vi "DRIVE_SPEED_CONTROL.vi"(4 "Time_Seconds":dbl, 5 "Speed PID":T2, 6 "Speed (PV)":dbl, 7 "SIMPLE_MOTOR_FF":T1 {"KnInv" format="%13.4f"; "Ka" format="%13.4f"; "Kv" format="%13.4f"; "Ks" format="%13.4f"}, 9 "Speed Target (SP)":dbl, 10 "Max SP Rate":dbl, 11 "Max Speed Ft/Sec":dbl) -> (0 "FeedForward":dbl, 1 "SpeedDmdAccel":dbl, 2 "SpeedDmd":dbl, 3 "CO-ControlOutput":dbl)   [LabVIEW 2019]
uses:
  DRIVE_PID_TUNING.ctl
  <vilib>/Rock Robotics/WPI/ThirdParty/JAS_Junk/TrajLib/TypeDef/SIMPLE_MOTOR_FF.ctl
  <vilib>/Rock Robotics/WPI/ThirdParty/JAS_Junk/TrajLib/SlewRateLimiter_New.vi
  <vilib>/Rock Robotics/WPI/ThirdParty/JAS_Junk/TrajLib/SlewRateLimiter_Reset.vi
  <vilib>/Rock Robotics/WPI/ThirdParty/JAS_Junk/TrajLib/SlewRateLimiter_Calculate.vi
  <vilib>/Rock Robotics/WPI/ThirdParty/JAS_Junk/TrajLib/SlewRateLimiter_SetRate.vi
  <vilib>/Rock Robotics/WPI/ThirdParty/JAS_Junk/TrajLib/PIDController_AtSetpoint.vi
  <vilib>/Rock Robotics/WPI/ThirdParty/JAS_Junk/TrajLib/PIDController_SetPIDF.vi
  <vilib>/Rock Robotics/WPI/ThirdParty/JAS_Junk/TrajLib/PIDController_SetDerivativeFilter.vi
  <vilib>/Rock Robotics/WPI/ThirdParty/JAS_Junk/TrajLib/PIDController_SetIntegratorRange.vi
  <vilib>/Rock Robotics/WPI/ThirdParty/JAS_Junk/TrajLib/PIDController_SetTolerancePandV.vi
  <vilib>/Rock Robotics/WPI/ThirdParty/JAS_Junk/TrajLib/PIDController_DisableContinousInput.vi
  <vilib>/Rock Robotics/WPI/ThirdParty/JAS_Junk/TrajLib/PIDController_EnableContinousInput.vi
  <vilib>/Rock Robotics/WPI/ThirdParty/JAS_Junk/TrajLib/PIDController_Reset.vi
  <vilib>/Rock Robotics/WPI/ThirdParty/JAS_Junk/TrajLib/PIDController_New.vi
  <vilib>/Rock Robotics/WPI/ThirdParty/JAS_Junk/TrajLib/PIDController_SetOutputLimits.vi
  <vilib>/Rock Robotics/WPI/ThirdParty/JAS_Junk/TrajLib/PIDController_NewPeriod.vi
  <vilib>/Rock Robotics/SystemInterfaces/NetworkCommunication/NetComm_UsageReport_report.vi
  <vilib>/Rock Robotics/WPI/ThirdParty/JAS_Junk/TrajLib/Util_GetTime.vi
  <vilib>/Rock Robotics/WPI/ThirdParty/JAS_Junk/TrajLib/Util_LibraryGlobals.vi
  <vilib>/Rock Robotics/WPI/ThirdParty/JAS_Junk/TrajLib/PIDController_AdvCalculate_FF_Sp_Pv.vi
  <vilib>/Rock Robotics/WPI/ThirdParty/JAS_Junk/TrajLib/Trajectory_Library.lvlib
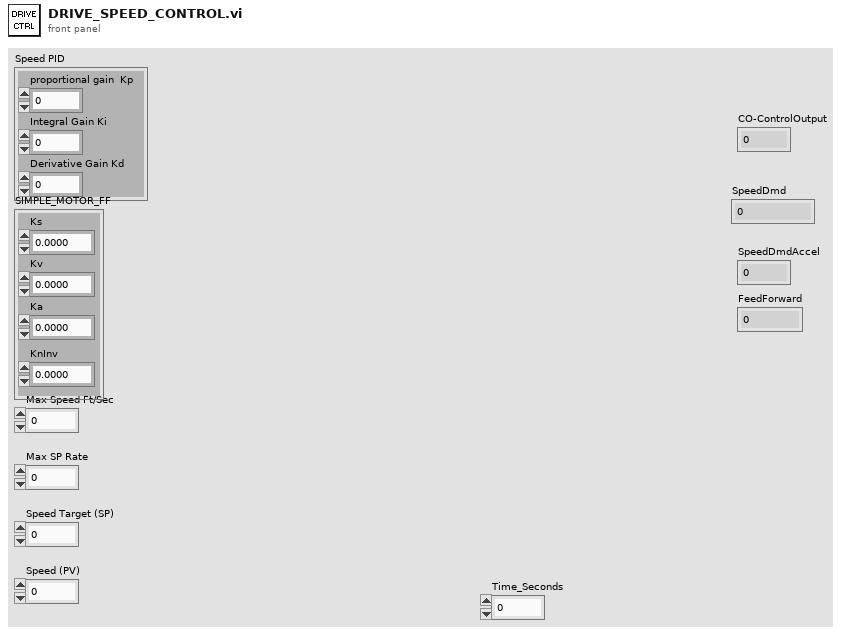
[diagram p1: front panel]
types:
  T1 = typedef "Trajectory_Library.lvlib/SIMPLE_MOTOR_FF.ctl" = cluster{"Ks":dbl, "Kv":dbl, "Ka":dbl, "KnInv":dbl}
  T2 = typedef "DRIVE_PID_TUNING.ctl" = cluster{"proportional gain  Kp":dbl, "Integral Gain Ki":dbl, "Derivative Gain Kd":dbl}
  T3 = typedef "Trajectory_Library.lvlib/PID_ADV_TUNING.ctl" = cluster{"Kf":dbl, "Kp":dbl, "Ki":dbl, "Kd":dbl, "MaximumIntegral":dbl, "MinimumIntegral":dbl, "Filter Derivative":bool}
  T4 = typedef "Trajectory_Library.lvlib/PID_ADV_LIMITS.ctl" = cluster{"MaxInput":dbl, "MinInput":dbl, "Continuous":bool, "MaxOutput":dbl, "MinOutput":dbl}
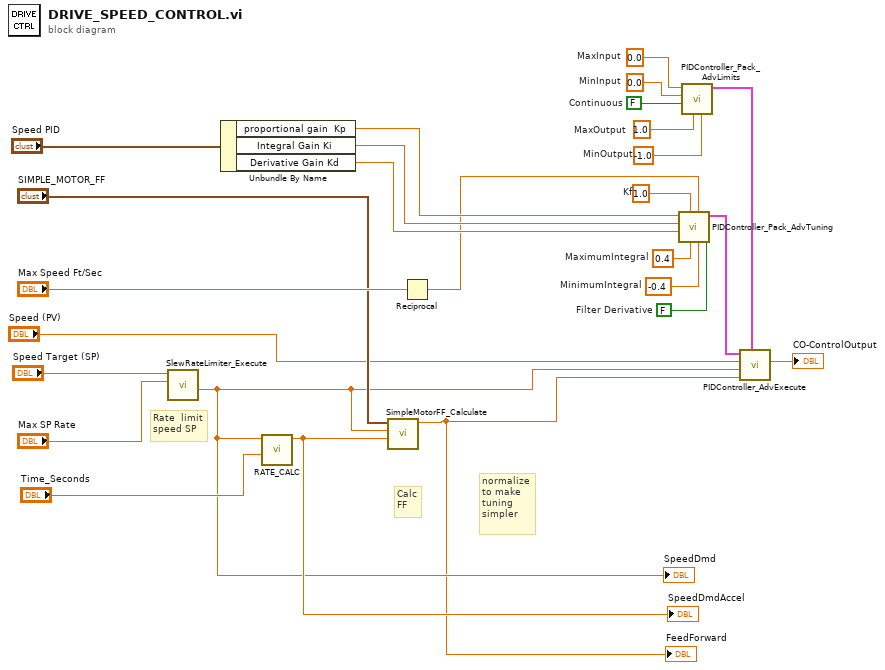
[diagram p0: block diagram]
diagram:
  w11 = 1.0  # Kf
  w12 = 0.4  # MaximumIntegral
  w13 = -0.4  # MinimumIntegral
  w14 = FALSE  # Filter Derivative
  w16 = 0.0  # MinInput
  w17 = FALSE  # Continuous
  w18 = 1.0  # MaxOutput
  w15 = -1.0  # MinOutput
  w19 = 0.0  # MaxInput
  # "Calc\nFF"
  # "Rate  limit\nspeed SP"
  # "normalize\nto make\ntuning\nsimpler"
  n1 = call <vilib>:"SlewRateLimiter_Execute.vi"("PositiveRate"="Max SP Rate", "Input"="Speed Target (SP)") -> ("Output"=w2:dbl)  [unwired: 8 in, 1 out]
  "SpeedDmd" <- w2
  n2 = Unbundle By Name("Speed PID") -> ("proportional gain  Kp"=w23:dbl, "Integral Gain Ki"=w24:dbl, "Derivative Gain Kd"=w25:dbl)
  n3 = call "RATE_CALC.vi"("Time"="Time_Seconds", "Input"=w2) -> ("Output"=w9:dbl)  [unwired: 9 in]
  "SpeedDmdAccel" <- w9
  n4 = call <vilib>:"SimpleMotorFF_Calculate.vi"("Accel"=w9, "Vel Sp"=w2, "SIMPLE_MOTOR_FF"="SIMPLE_MOTOR_FF") -> ("FeedForward"=w1:dbl)  [unwired: 8 in]
  "FeedForward" <- w1
  n5 = Reciprocal(x="Max Speed Ft/Sec") -> (1/x=w4:dbl)
  n6 = call <vilib>:"PIDController_Pack_AdvTuning.vi"("Filter Derivative"=w14, "MinimumIntegral"=w13, "Kn"=w4, "MaximumIntegral"=w12, "Kf"=w11, "Kd"=w25, "Ki"=w24, "Kp"=w23) -> ("Adv PID Tuning"=w20:T3)  [unwired: 3 in]
  n7 = call <vilib>:"PIDController_Pack_AdvLimits.vi"("MinOutput"=w15, "MaxOutput"=w18, "Continuous"=w17, "MinInput"=w16, "MaxInput"=w19) -> ("Adv PID Limits"=w21:T4)  [unwired: 6 in]
  n8 = call <vilib>:"PIDController_AdvExecute.vi"("Adv PID Limits"=w21, "FF-FeedForward"=w1, "SP-SetPoint"=w2, "PV-Measurement"="Speed (PV)", "Adv PID Tuning"=w20) -> ("CO-ControlOutput"=→"CO-ControlOutput":dbl)  [unwired: 4 in, 2 out]
